vi "dx Grab simple.vi"() -> ()   [LabVIEW 2020]
doc: "The Grab with Bayer Decoding VI acquires images continuously and displays the decoded Bayer image as an RGB image in an image control on the front panel. \n\nIMAQ Create Bayer LUT configures the gains to apply to the color planes. Refer to the Bayer decoding documentation in the White Balancing Utility for more information about setting the appropriate gains. Initialize the LUT only once to minimize decoding time. IMAQ Bayer Color Decode decodes a monochrome image to create the RGB image. An image control displays the RGB image on the front panel. After exiting the loop, IMAQ Extract Buffer releases the last extracted buffer. IMAQ Close releases resources associated with the acquisition, and IMAQ Dispose frees the buffers used for acquisition and Bayer decoding."
uses:
  <vilib>/vision/driver/NI_Vision_Acquisition_Software.lvlib
panel:
  out "error out":errorcluster
  out "Image":T1(plugin-control)
  out "Image Pixels (U32)":u32[][](array[numeric])
  out "save error":errorcluster
  in  "milliseconds to wait":u32=200
  in  "File Path":path=path "c:/temp"
  in  "Save":bool
  out "Buffer Number":u32
  in  "Camera Name":refnum<k21> caption="IMAQdx Session"
  in  "Stop":bool
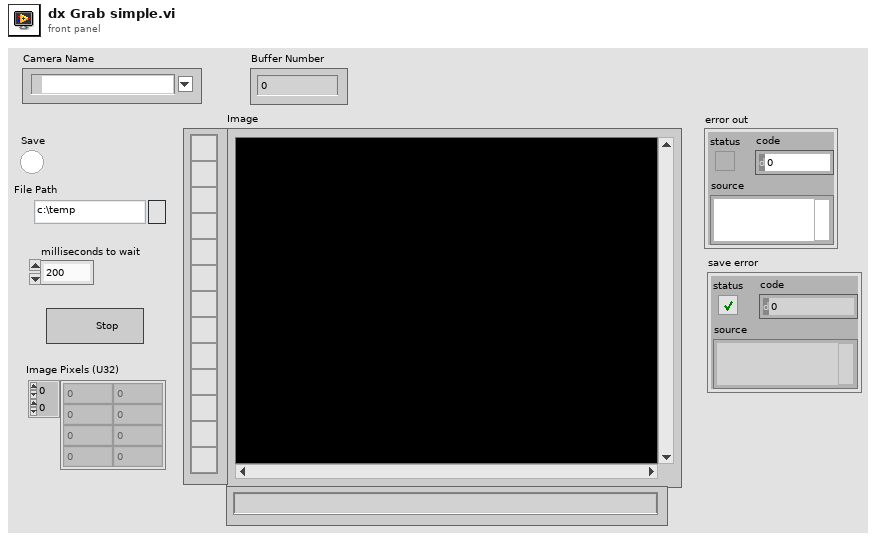
[diagram p1: front panel]
types:
  T1 = typedef "IMAQ Image.ctl" = refnum<image>
  T2 = typedef "Image Type" = u32
  T3 = typedef "IMAQdx.ctl" = refnum<k21>
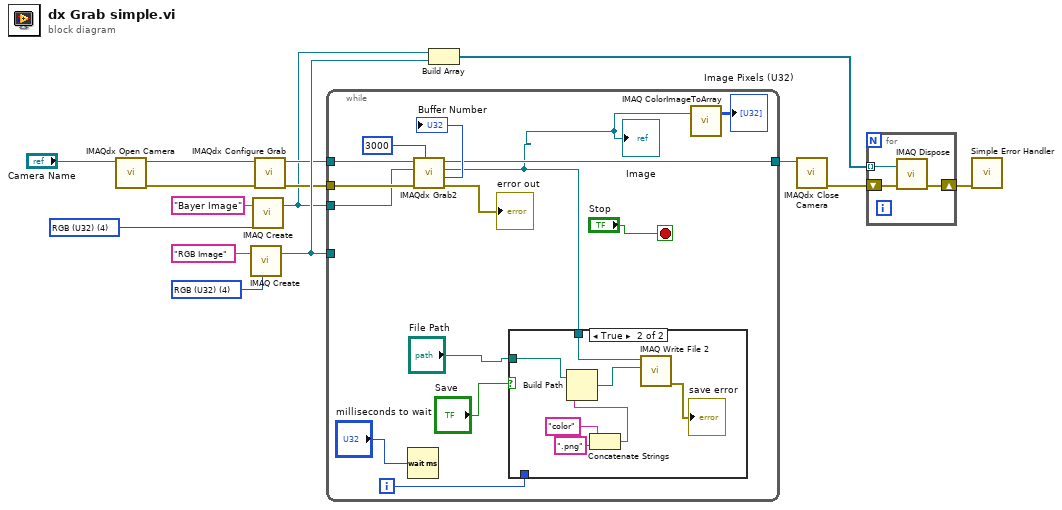
[diagram p0: block diagram]
diagram:
  w1 = T2 4 items=["Grayscale (U8)", "Grayscale (I16)", "Grayscale (SGL)", "Complex (CSG)", "RGB (U32)", "HSL (U32)", "RGB (U64)", "Grayscale (U16)"] ("Image Type")
  w10 = T2 4 items=["Grayscale (U8)", "Grayscale (I16)", "Grayscale (SGL)", "Complex (CSG)", "RGB (U32)", "HSL (U32)", "RGB (U64)", "Grayscale (U16)"] ("Image Type")
  n1 = call <vilib>:"IMAQdx Open Camera.vi"("Session In"="Camera Name") -> ("error out"=w2:errorcluster, "Session Out"=w3:T3)  [unwired: 9 in]
  n2 = call "IMAQ Create"("Image Name"="RGB Image", "Image Type"=w10) -> ("New Image"=w9:T1)  [unwired: 2 in, 2 out]
  n3 = call "IMAQ Create"("Image Name"="Bayer Image", "Image Type"=w1) -> ("New Image"=w5:T1)  [unwired: 2 in, 2 out]
  n4 = call <vilib>:"IMAQdx Configure Grab.vi"("error in"=w2, "Session In"=w3) -> ("error out"=w8:errorcluster, "Session Out"=w7:T3)  [unwired: 8 in]
  n5 = while {
    tunnel: w9 -> [_]
    tunnel: [w21] -> w4
    tunnel: w7 -> [w29]
    tunnel: w8 -> [w28]
    tunnel: w5 -> [w26]
    i -> [w23]
    stop <- "Stop" stop-if-true
    n6 = Wait (ms)(milliseconds to wait="milliseconds to wait") -> ()  [unwired: 1 out]
    n7 = call <vilib>:"IMAQdx Grab2.vi"("Timeout (ms)"=3000, "error in"=w28, "Image In"=w26, "Session In"=w29) -> ("error out"=→"error out":errorcluster, "Buffer Number Out"=→"Buffer Number":u32, "Image Out"=w19:T1, "Session Out"=w21:T3)  [unwired: 4 in]
    "Image" <- w19
    n8 = case shown="True" "Save" {
      tunnel: "File Path" -> [_ w36]
      tunnel: w23 -> [_ _]
      tunnel: w19 -> [_ w31]
      frame False {
      }
      frame True {
        n9 = Concatenate Strings("color" ("string"), ".png" ("string")) -> (w34:string)
        n10 = Build Path(base path=w36, name or relative path=w34) -> (appended path=w33:path)
        n11 = call-poly "IMAQ Write File 2"("File Path"=w33, "Image"=w31) -> ("error out"=→"save error":errorcluster)  [unwired: 8 in, 1 out]
      }
    }
    n12 = call "IMAQ ColorImageToArray"("Image"=w19) -> ("Image Pixels (U32)"=→"Image Pixels (U32)":u32[][])  [unwired: 3 in, 2 out]
  }
  n13 = Build Array(w5, w9) -> (w13:T1[])
  n14 = call <vilib>:"IMAQdx Close Camera.vi"("Session In"=w4) -> ("error out"=w12:errorcluster)  [unwired: 10 in]
  n15 = for {
    tunnel: w13 -> [w39] mode=indexing
    shift-right: [w37] -> w11
    shift-left: w12 -> [w38]
    n16 = call "IMAQ Dispose"("Image"=w39, "error in (no error)"=w38) -> ("error out"=w37:errorcluster)  [unwired: 1 in, 3 out]
  }
  n17 = call <vilib>:"Simple Error Handler.vi"("error in (no error)"=w11) -> ()  [unwired: 1 in, 8 out]
